vi "IED_Status_0 Entry Timeout.vi"(11 "SCADA in":refnum<class "EMS.lvclass">) -> ()   [LabVIEW 2018, in "EMS Core.lvlib" / "EMS.lvclass"]
uses:
  EMS.lvclass
  C:/Users/Administrator/Desktop/LabVIEW EMS/EMS Generic Actor/EMS Generic/EMS Generic.lvclass
  <vilib>/ORNL/CSEISMIC DDS/CSEISMIC DDS Base/Data Types/Controls/Timestamp.ctl
  EMS Generic Actor/EMS Generic/EMS Generic.lvclass/EMS Generic.ctl
  <vilib>/ORNL/CSEISMIC DDS/CSEISMIC DDS Base/Data Types/IED_Status.ctl
  <vilib>/ORNL/CSEISMIC DDS/CSEISMIC DDS Base/Data Types/Controls/DeviceID.ctl
  <vilib>/ORNL/CSEISMIC DDS/CSEISMIC DDS Base/CSEISMIC DDS.lvclass
  Utilities/Status Messaging.llb/Status Messaging.lvlib
  EMS Generic Actor/EMS Generic/EMS Generic.lvclass
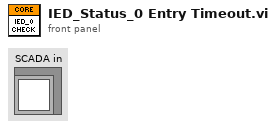
[diagram p1: front panel]
types:
  T1 = typedef "CSEISMIC DDS.lvlib/CSEISMIC DDS.lvclass/Timestamp.ctl" = cluster{"Seconds":u64, "Remainder":u64}
  T2 = typedef "EMS Generic Actor.lvlib/EMS Generic.lvclass/Data Type DVRs.ctl" = cluster{"IED_Status":refnum<data-value>, "IED_Status_0":refnum<data-value>, "DER_Measurement":refnum<data-value>, "DER_Info":refnum<data-value>, "DER_Status":refnum<data-value>, "ES_Measurement":refnum<data-value>, "ES_Info":refnum<data-value>, "PV_Info":refnum<data-value>, "SmartRelay_Info":refnum<data-value>, "SmartRelay_Measurement":refnum<data-value>, "Meter_Info":refnum<data-value>, "Meter_Measurement":refnum<data-value>, "HVAC_Status":refnum<data-value>, "HVAC_Measurement":refnum<data-value>, "PriceData_RealTime":refnum<data-value>, "PriceData_Demand":refnum<data-value>, "PriceData_Energy":refnum<data-value>, "ForecastData_Long":refnum<data-value>, "ForecastData_Short":refnum<data-value>, "DER_Control":refnum<data-value>, "DER_SetPointF":refnum<data-value>, "DER_SetPointP":refnum<data-value>, "DER_SetPointQ":refnum<data-value>, "DER_SetPointPF":refnum<data-value>, "DER_SetPointV":refnum<data-value>, "PV_setCurtailment":refnum<data-value>, "PV_setRampRate":refnum<data-value>, "Relay_Control":refnum<data-value>, "Load_Control":refnum<data-value>, "HVAC_Control":refnum<data-value>, "Generator_Info":refnum<data-value>, "ForecastData_Long_Backup":refnum<data-value>, "PriceData_RealTime_Backup":refnum<data-value>}
  T3 = typedef "CSEISMIC DDS.lvlib/CSEISMIC DDS.lvclass/DeviceID.ctl" = string
  T4 = typedef "CSEISMIC DDS.lvlib/CSEISMIC DDS.lvclass/IED_Status.ctl" = cluster{"DeviceID":T3, "Timestamp":T1, "MicrogridID":u8, "Active":bool, "Inactive":bool, "Error":i32, "Fault":bool, "ErrorString":string}
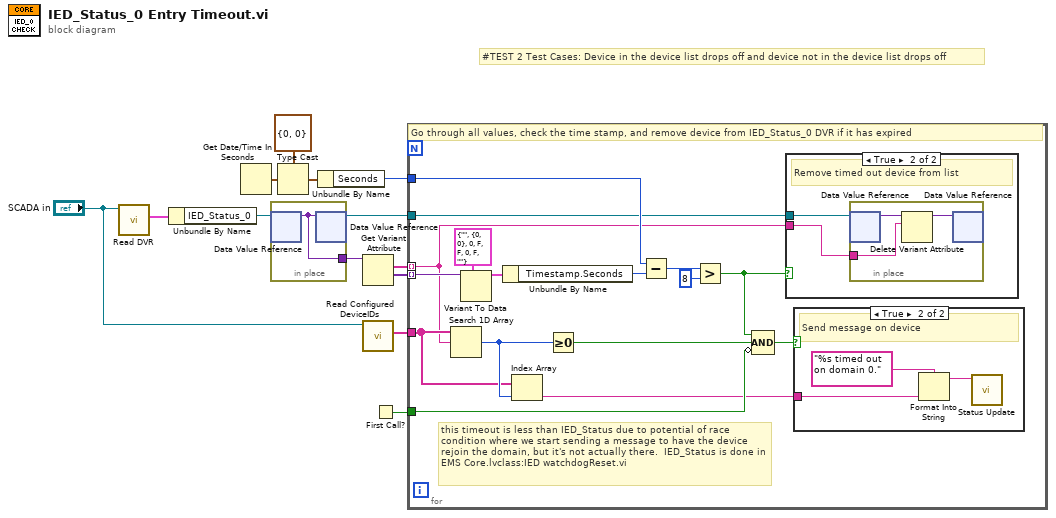
[diagram p0: block diagram]
diagram:
  # "#TEST 2 Test Cases: Device in the device list drops off and device not in the device list drops off"
  n1 = call "Read DVR.vi"("EMS Generic in"="SCADA in") -> ("DVR"=w13:T2)  [unwired: 9 in, 1 out]
  n2 = Unbundle By Name(w13) -> ("IED_Status_0"=w1:refnum<data-value>)
  n3 = Get Date/Time In Seconds() -> (seconds since 1Jan1904=w8:timestamp)
  n4 = in-place {
    in-place-border: [w14] -> w3
    n5 = in-place-dvr #1(w1) -> (w14:variant)  [unwired: 1 out]
    n6 = in-place-dvr #1(w14) -> (w2:refnum<data-value>)  [unwired: 1 out]
  }
  n7 = Type Cast(type=T1 {"Seconds"=0, "Remainder"=0} ("Timestamp"), x=w8) -> (*(type *) &x=w6:T1)
  n8 = Unbundle By Name(w6) -> ("Seconds"=w9:u64)
  n9 = Get Variant Attribute(Variant=w3) -> (names=w4:string[], values=w5:variant[])  [unwired: 3 in, 2 out]
  n10 = call "Read Configured DeviceIDs.vi"("EMS Generic in"="SCADA in") -> ("DeviceIDs"=w10:T3[])  [unwired: 8 in, 2 out]
  n11 = First Call?() -> (First Call?: T/F=w11:bool)
  n12 = for {
    tunnel: w5 -> [w21] mode=indexing
    tunnel: w4 -> [w16] mode=indexing
    tunnel: w2 -> [w22]
    tunnel: w9 -> [w26]
    tunnel: w10 -> [w19]
    tunnel: w11 -> [w23]
    # "this timeout is less than IED_Status due to potential of race condition where we start sending a message to have the device rejoin the domain, but it's not actually there.  IED_Status is done in EMS Core.lvclass:IED watchdogReset.vi"
    # "Go through all values, check the time stamp, and remove device from IED_Status_0 DVR if it has expired"
    n13 = Search 1D Array(1D array=w19, element=w16) -> (index of element=w20:i32)  [unwired: 1 in]
    n14 = Variant To Data(type=T4 {"DeviceID"="", "Timestamp"={"Seconds"=0, "Remainder"=0}, "MicrogridID"=0, "Active"=FALSE, "Inactive"=FALSE, "Error"=0, "Fault"=FALSE, "ErrorString"=""} ("IED_Status"), Variant=w21) -> (data=w30:T4)  [unwired: 1 in, 1 out]
    n15 = Unbundle By Name(w30) -> ("Timestamp.Seconds"=w29:u64)
    n16 = Index Array(array=w19, index=w20) -> (element=w18:T3)
    n17 = Greater Or Equal To 0?(x=w20) -> (x >= 0?=w25:bool)
    n18 = Subtract(x=w26, y=w29) -> (x-y=w15:u64)
    n19 = Greater?(x=w15, y=u64 8) -> (0:w17:bool)
    n20 = Compound Arithmetic op=AND(w17, w25, invert w23) -> (w24:bool)
    n21 = case shown="True" w17 {
      tunnel: w22 -> [_ w32]
      tunnel: w16 -> [_ w31]
      frame False {
      }
      frame True {
        # "Remove timed out device from list"
        n22 = in-place {
          in-place-border: w31 -> [w34]
          n23 = in-place-dvr #2(w32) -> (w35:variant)  [unwired: 1 out]
          n24 = Delete Variant Attribute(6:w34, 7:w35) -> (3:w33:variant)  [unwired: 1 in, 2 out]
          n25 = in-place-dvr #2(w33) -> ()  [unwired: 2 out]
        }
      }
    }
    n26 = case shown="True" w24 {
      tunnel: w18 -> [_ w37]
      frame False {
        # "Do nothing"
      }
      frame True {
        # "Send message on device"
        n27 = Format Into String(format string="%s timed out on domain 0.", w37) -> (resulting string=w36:string)  [unwired: 2 in, 1 out]
        n28 = call "Status Update.vi"("Status Update"=w36) -> ()  [unwired: 9 in, 2 out]
      }
    }
  }
